vi "MPU_Stick_Generate_Emulator_Data.vi"() -> ()   [LabVIEW 2017]
uses:
  <vilib>/Utility/file.llb/Write Delimited Spreadsheet (string).vi
panel:
  in  "Step time (ms)":dbl=100.0
  in  "Number of samples":i32=100
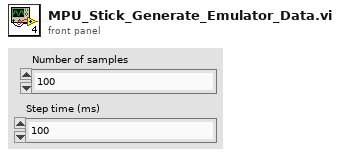
[diagram p1: front panel]
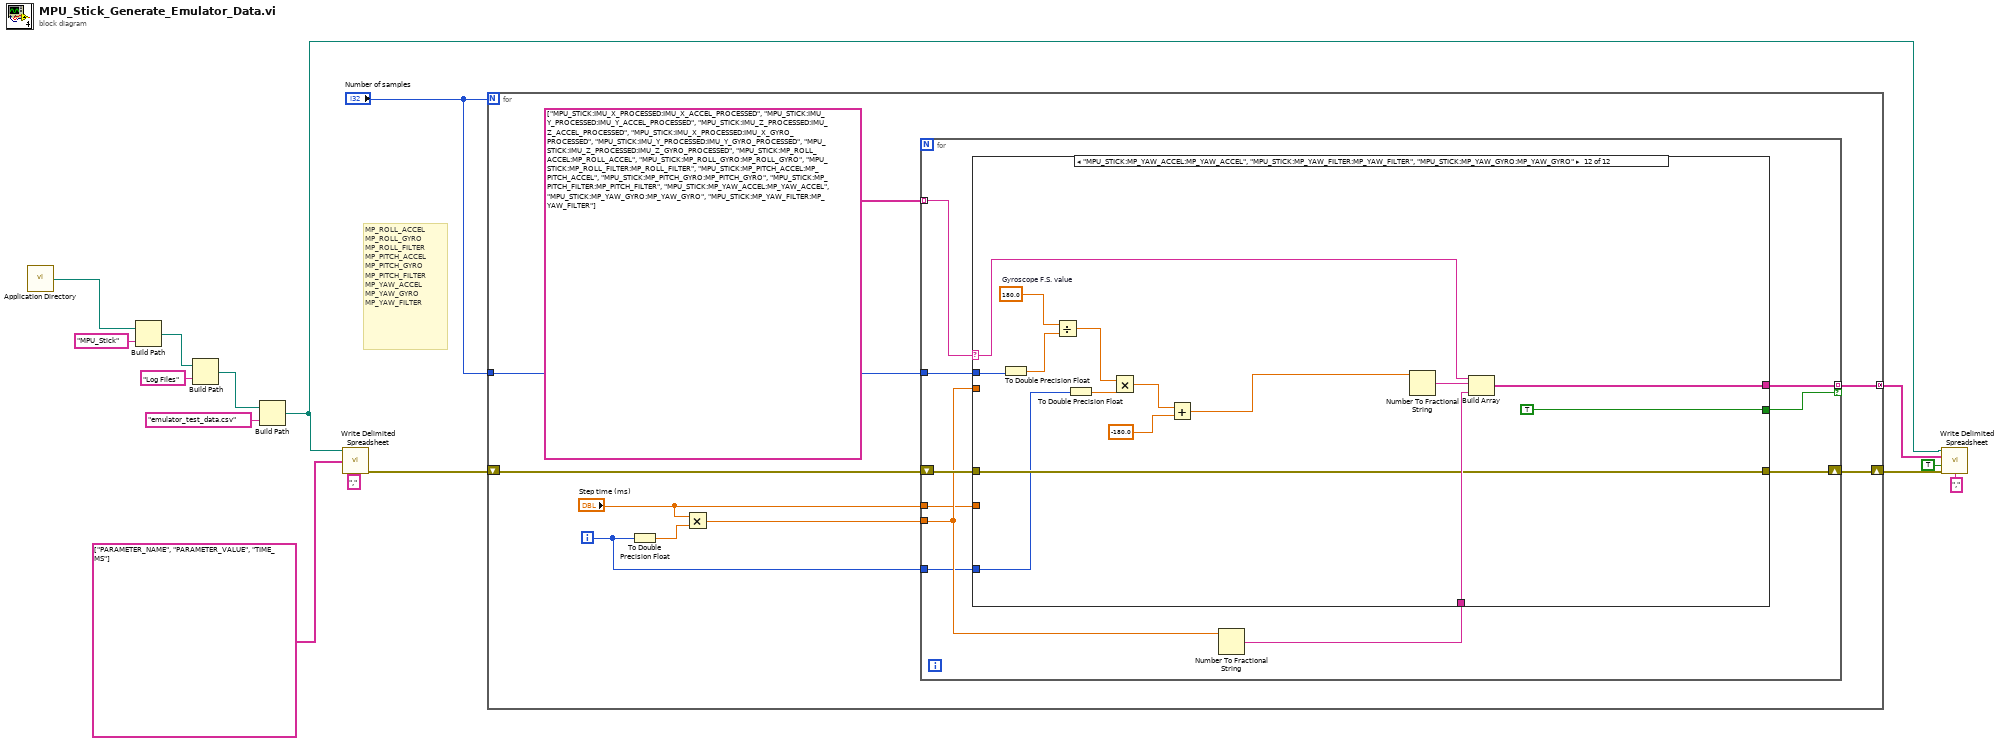
[diagram p0: block diagram]
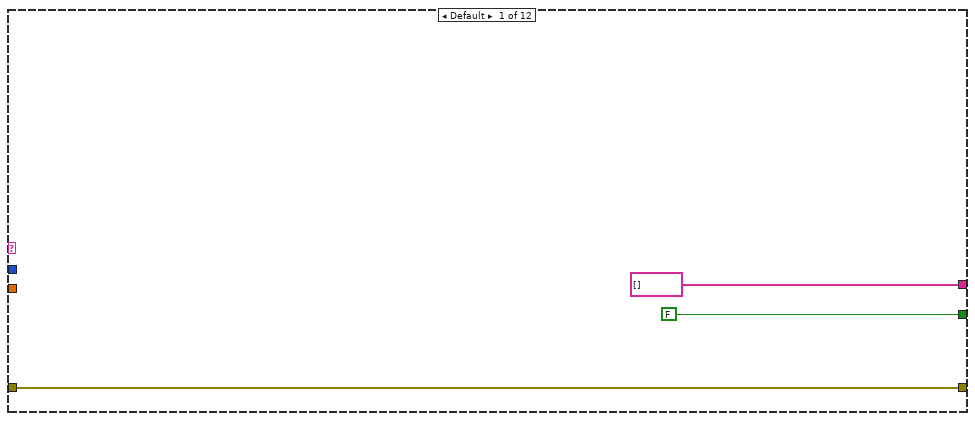
[diagram p2: hidden frame]
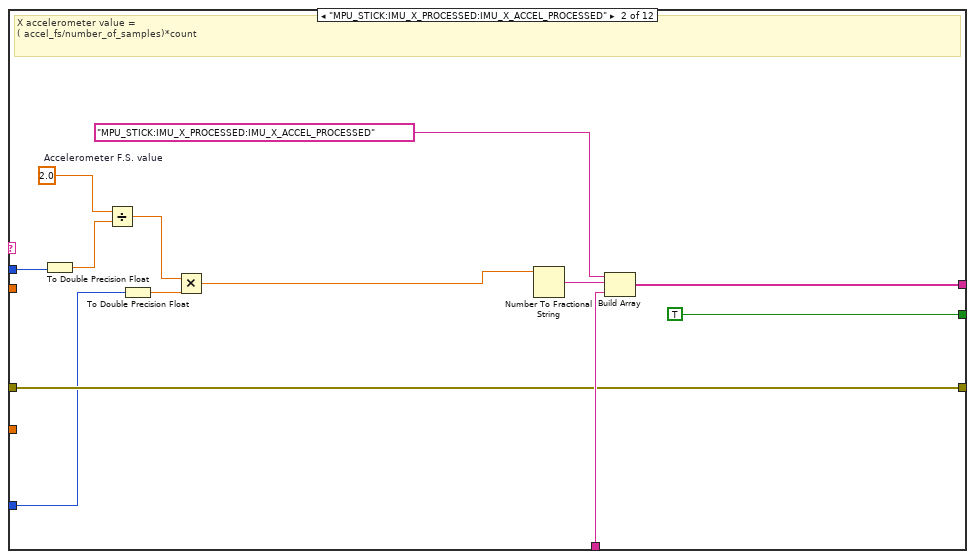
[diagram p3: hidden frame]
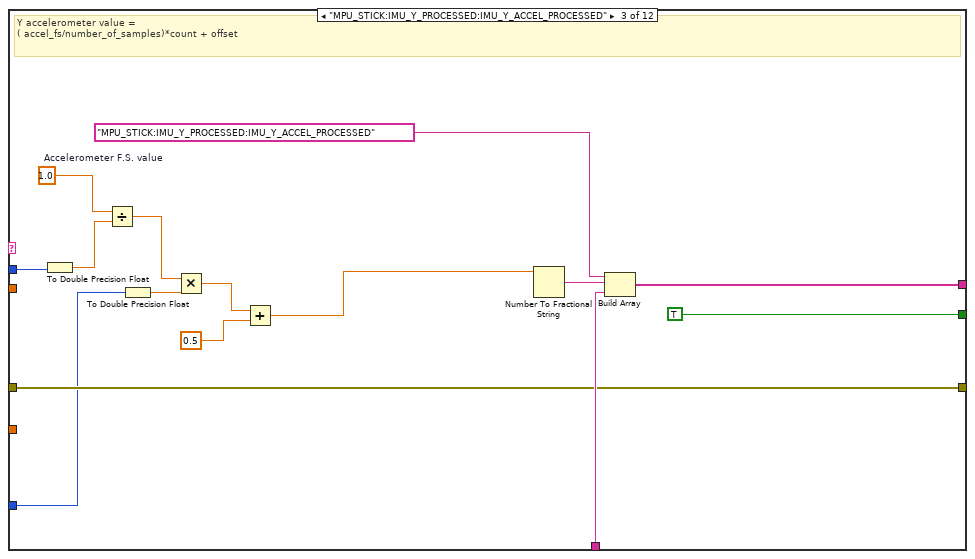
[diagram p4: hidden frame]
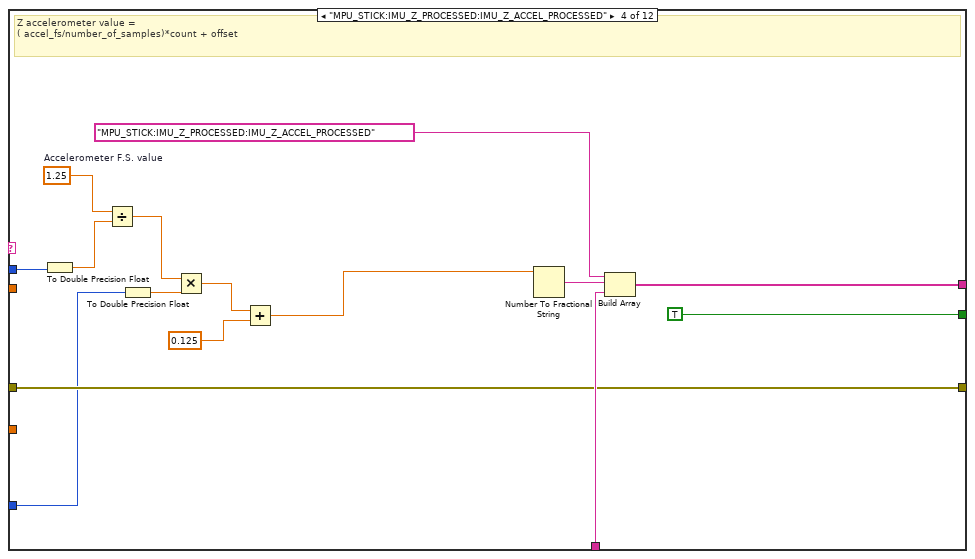
[diagram p5: hidden frame]
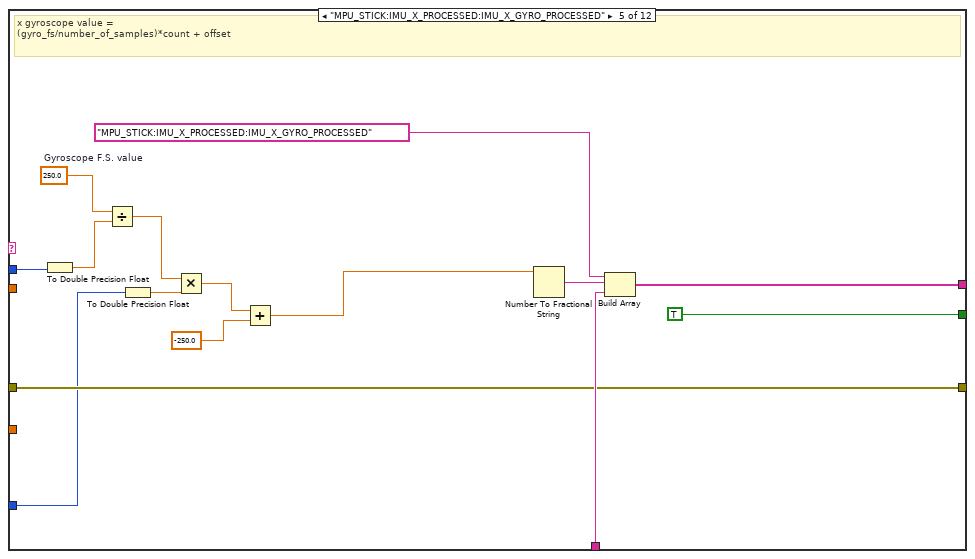
[diagram p6: hidden frame]
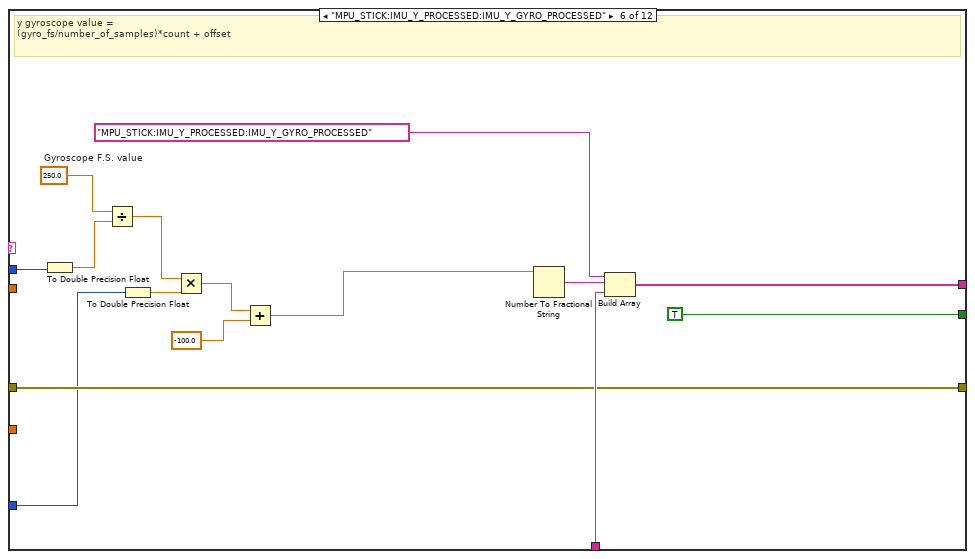
[diagram p7: hidden frame]
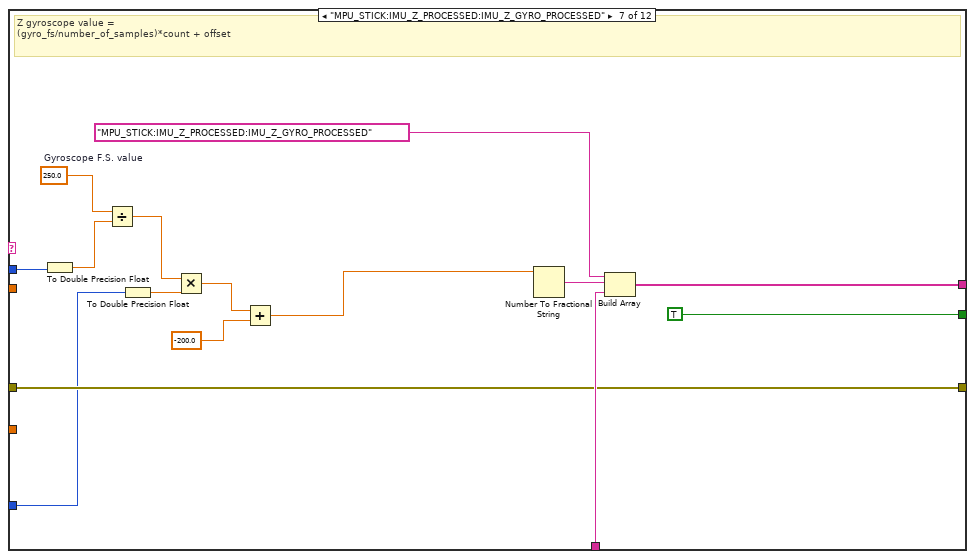
[diagram p8: hidden frame]
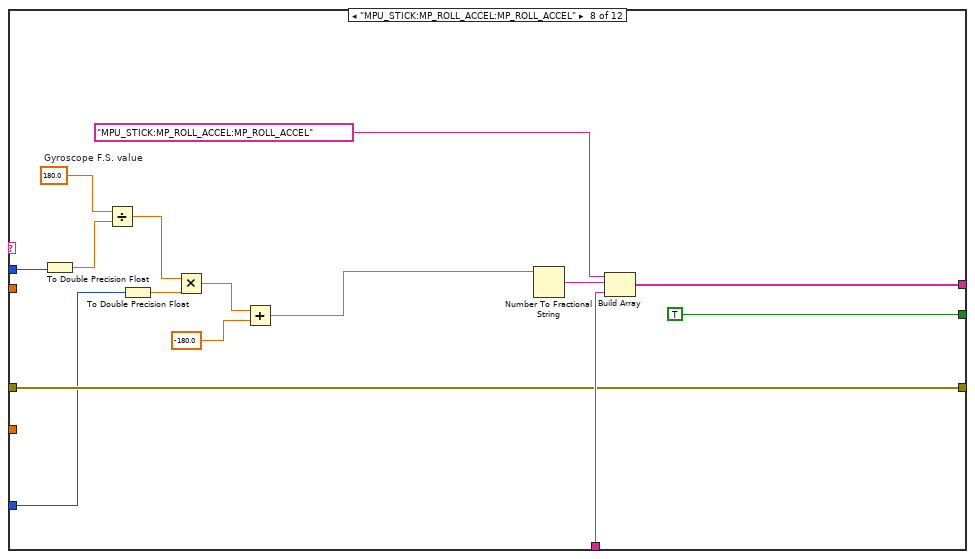
[diagram p9: hidden frame]
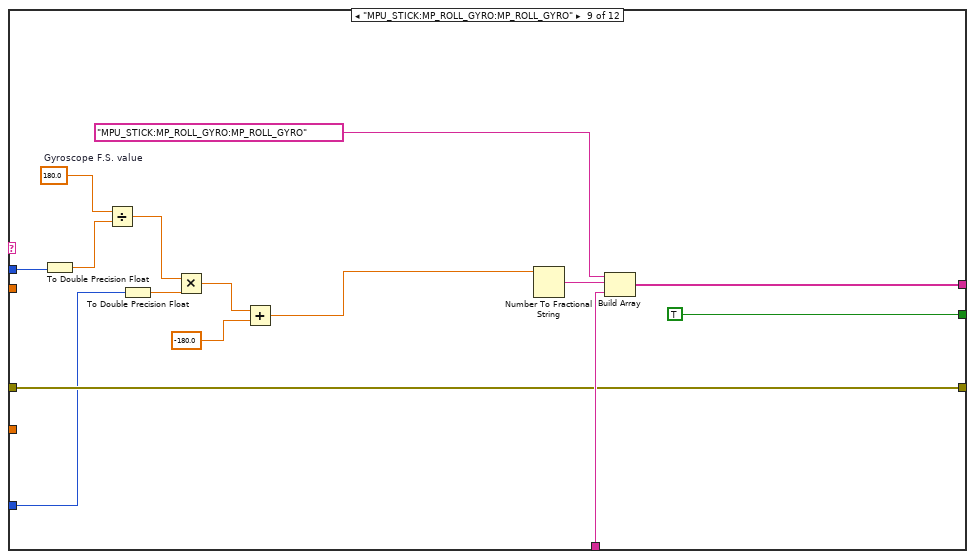
[diagram p10: hidden frame]
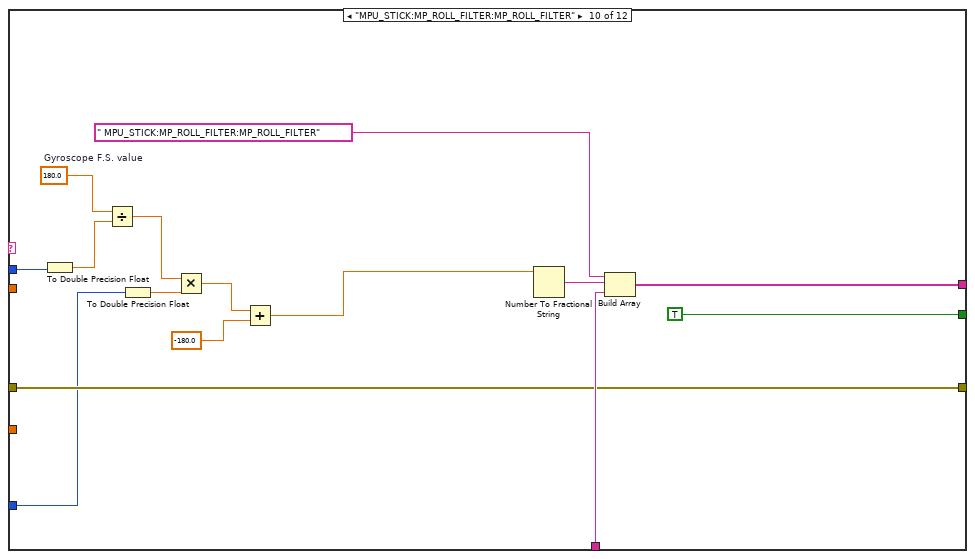
[diagram p11: hidden frame]
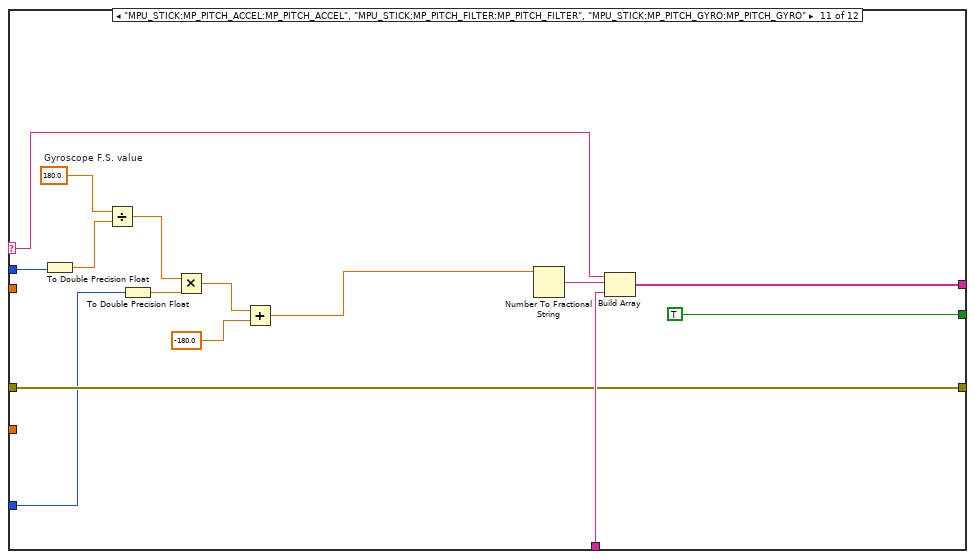
[diagram p12: hidden frame]
diagram:
  # "MP_ROLL_ACCEL\nMP_ROLL_GYRO\nMP_ROLL_FILTER\nMP_PITCH_ACCEL\nMP_PITCH_GYRO\nMP_PITCH_FILTER\nMP_YAW_ACCEL\nMP_YAW_GYRO\nMP_YAW_FILTER"
  n1 = call <vilib>:"Application Directory.vi"() -> ("Application Directory"=w10:path)
  n2 = Build Path(base path=w10, name or relative path="MPU_Stick") -> (appended path=w9:path)
  n3 = Build Path(base path=w9, name or relative path="Log Files") -> (appended path=w14:path)
  n4 = Build Path(base path=w14, name or relative path="emulator_test_data.csv") -> (appended path=w5:path)
  n5 = call-poly <vilib>:"Write Delimited Spreadsheet.vi"("file path (dialog if empty)"=w5, "1D data"=string[] ["PARAMETER_NAME", "PARAMETER_VALUE", "TIME_MS"], "delimiter (\\t)"="," ("delimiter (\\t)")) -> ("error out"=w7:errorcluster)  [unwired: 11 in, 1 out]
  n6 = for {
    N: "Number of samples" -> [_]
    shift-right: [w20] -> w6
    shift-left: w7 -> [w23]
    tunnel: [w17] -> w4 mode=concatenating
    tunnel: "Number of samples" -> [w16]
    i -> [w19]
    n7 = To Double Precision Float(number=w19) -> (double precision float=w22:dbl)
    n8 = Multiply(x="Step time (ms)", y=w22) -> (x*y=w21:dbl)
    n9 = for {
      tunnel: string[] ["MPU_STICK:IMU_X_PROCESSED:IMU_X_ACCEL_PROCESSED", "MPU_STICK:IMU_Y_PROCESSED:IMU_Y_ACCEL_PROCESSED", "MPU_STICK:IMU_Z_PROCESSED:IMU_Z_ACCEL_PROCESSED", "MPU_STICK:IMU_X_PROCESSED:IMU_X_GYRO_PROCESSED", "MPU_STICK:IMU_Y_PROCESSED:IMU_Y_GYRO_PROCESSED", "MPU_STICK:IMU_Z_PROCESSED:IMU_Z_GYRO_PROCESSED", "MPU_STICK:MP_ROLL_ACCEL:MP_ROLL_ACCEL", "MPU_STICK:MP_ROLL_GYRO:MP_ROLL_GYRO", "MPU_STICK:MP_ROLL_FILTER:MP_ROLL_FILTER", "MPU_STICK:MP_PITCH_ACCEL:MP_PITCH_ACCEL", "MPU_STICK:MP_PITCH_GYRO:MP_PITCH_GYRO", "MPU_STICK:MP_PITCH_FILTER:MP_PITCH_FILTER", "MPU_STICK:MP_YAW_ACCEL:MP_YAW_ACCEL", "MPU_STICK:MP_YAW_GYRO:MP_YAW_GYRO", "MPU_STICK:MP_YAW_FILTER:MP_YAW_FILTER"] -> [w33] mode=indexing
      tunnel: w21 -> [w31]
      shift-right: [w32] -> w20
      shift-left: w23 -> [w34]
      tunnel: w19 -> [w30]
      tunnel: "Step time (ms)" -> [w29]
      tunnel: [w27] -> w17 mode=indexing if=w26
      tunnel: w16 -> [w25]
      n10 = Number To Fractional String(number=w31) -> (F-format string=w28:string)  [unwired: 3 in]
      n11 = case shown="\"MPU_STICK:MP_YAW_ACCEL:MP_YAW_ACCEL\", \"MPU_STICK:MP_YAW_FILTER:MP_YAW_FILTER\", \"MPU_STICK:MP_YAW_GYRO:MP_YAW_GYRO\"" w33 {
        selector: w33 -> [_ _ _ _ _ _ _ _ _ _ w171 w186]
        tunnel: w34 -> [w37 w47 w62 w77 w92 w107 w122 w137 w152 w167 w183 w198]
        tunnel: [w37 w47 w62 w77 w92 w107 w122 w137 w152 w167 w183 w198] -> w32
        tunnel: w31 -> [_ _ _ _ _ _ _ _ _ _ _ _]
        tunnel: w30 -> [_ w40 w55 w70 w85 w100 w115 w130 w145 w160 w176 w191]
        tunnel: w29 -> [_ _ _ _ _ _ _ _ _ _ _ _]
        tunnel: w28 -> [_ w48 w63 w78 w93 w108 w123 w138 w153 w168 w184 w199]
        tunnel: [string[] [] w46 w61 w76 w91 w106 w121 w136 w151 w166 w182 w197] -> w27
        tunnel: [FALSE TRUE TRUE TRUE TRUE TRUE TRUE TRUE TRUE TRUE TRUE TRUE] -> w26
        tunnel: w25 -> [_ w43 w58 w73 w88 w103 w118 w133 w148 w163 w179 w194]
        frame Default {
        }
        frame "MPU_STICK:IMU_X_PROCESSED:IMU_X_ACCEL_PROCESSED" {
          w44 = 2.0  # Accelerometer F.S. value
          # "X accelerometer value =\n( accel_fs/number_of_samples)*count"
          n12 = To Double Precision Float(number=w43) -> (double precision float=w42:dbl)
          n13 = Divide(x=w44, y=w42) -> (x/y=w41:dbl)
          n14 = To Double Precision Float(number=w40) -> (double precision float=w39:dbl)
          n15 = Multiply(x=w41, y=w39) -> (x*y=w38:dbl)
          n16 = Number To Fractional String(number=w38) -> (F-format string=w50:string)  [unwired: 3 in]
          n17 = Build Array("MPU_STICK:IMU_X_PROCESSED:IMU_X_ACCEL_PROCESSED", w50, w48) -> (w46:string[])
        }
        frame "MPU_STICK:IMU_Y_PROCESSED:IMU_Y_ACCEL_PROCESSED" {
          w59 = 1.0  # Accelerometer F.S. value
          # "Y accelerometer value =\n( accel_fs/number_of_samples)*count + offset"
          n18 = To Double Precision Float(number=w58) -> (double precision float=w57:dbl)
          n19 = Divide(x=w59, y=w57) -> (x/y=w56:dbl)
          n20 = To Double Precision Float(number=w55) -> (double precision float=w54:dbl)
          n21 = Multiply(x=w56, y=w54) -> (x*y=w53:dbl)
          n22 = Add(x=w53, y=0.5) -> (x+y=w51:dbl)
          n23 = Number To Fractional String(number=w51) -> (F-format string=w65:string)  [unwired: 3 in]
          n24 = Build Array("MPU_STICK:IMU_Y_PROCESSED:IMU_Y_ACCEL_PROCESSED", w65, w63) -> (w61:string[])
        }
        frame "MPU_STICK:IMU_Z_PROCESSED:IMU_Z_ACCEL_PROCESSED" {
          w74 = 1.25  # Accelerometer F.S. value
          # "Z accelerometer value =\n( accel_fs/number_of_samples)*count + offset"
          n25 = To Double Precision Float(number=w73) -> (double precision float=w72:dbl)
          n26 = Divide(x=w74, y=w72) -> (x/y=w71:dbl)
          n27 = To Double Precision Float(number=w70) -> (double precision float=w69:dbl)
          n28 = Multiply(x=w71, y=w69) -> (x*y=w68:dbl)
          n29 = Add(x=w68, y=0.125) -> (x+y=w66:dbl)
          n30 = Number To Fractional String(number=w66) -> (F-format string=w80:string)  [unwired: 3 in]
          n31 = Build Array("MPU_STICK:IMU_Z_PROCESSED:IMU_Z_ACCEL_PROCESSED", w80, w78) -> (w76:string[])
        }
        frame "MPU_STICK:IMU_X_PROCESSED:IMU_X_GYRO_PROCESSED" {
          w89 = 250.0  # Gyroscope F.S. value
          # "x gyroscope value =\n(gyro_fs/number_of_samples)*count + offset"
          n32 = To Double Precision Float(number=w88) -> (double precision float=w87:dbl)
          n33 = Divide(x=w89, y=w87) -> (x/y=w86:dbl)
          n34 = To Double Precision Float(number=w85) -> (double precision float=w84:dbl)
          n35 = Multiply(x=w86, y=w84) -> (x*y=w83:dbl)
          n36 = Add(x=w83, y=-250.0) -> (x+y=w81:dbl)
          n37 = Number To Fractional String(number=w81) -> (F-format string=w95:string)  [unwired: 3 in]
          n38 = Build Array("MPU_STICK:IMU_X_PROCESSED:IMU_X_GYRO_PROCESSED", w95, w93) -> (w91:string[])
        }
        frame "MPU_STICK:IMU_Y_PROCESSED:IMU_Y_GYRO_PROCESSED" {
          w104 = 250.0  # Gyroscope F.S. value
          # "y gyroscope value =\n(gyro_fs/number_of_samples)*count + offset"
          n39 = To Double Precision Float(number=w103) -> (double precision float=w102:dbl)
          n40 = Divide(x=w104, y=w102) -> (x/y=w101:dbl)
          n41 = To Double Precision Float(number=w100) -> (double precision float=w99:dbl)
          n42 = Multiply(x=w101, y=w99) -> (x*y=w98:dbl)
          n43 = Add(x=w98, y=-100.0) -> (x+y=w96:dbl)
          n44 = Number To Fractional String(number=w96) -> (F-format string=w110:string)  [unwired: 3 in]
          n45 = Build Array("MPU_STICK:IMU_Y_PROCESSED:IMU_Y_GYRO_PROCESSED", w110, w108) -> (w106:string[])
        }
        frame "MPU_STICK:IMU_Z_PROCESSED:IMU_Z_GYRO_PROCESSED" {
          w119 = 250.0  # Gyroscope F.S. value
          # "Z gyroscope value =\n(gyro_fs/number_of_samples)*count + offset"
          n46 = To Double Precision Float(number=w118) -> (double precision float=w117:dbl)
          n47 = Divide(x=w119, y=w117) -> (x/y=w116:dbl)
          n48 = To Double Precision Float(number=w115) -> (double precision float=w114:dbl)
          n49 = Multiply(x=w116, y=w114) -> (x*y=w113:dbl)
          n50 = Add(x=w113, y=-200.0) -> (x+y=w111:dbl)
          n51 = Number To Fractional String(number=w111) -> (F-format string=w125:string)  [unwired: 3 in]
          n52 = Build Array("MPU_STICK:IMU_Z_PROCESSED:IMU_Z_GYRO_PROCESSED", w125, w123) -> (w121:string[])
        }
        frame "MPU_STICK:MP_ROLL_ACCEL:MP_ROLL_ACCEL" {
          w134 = 180.0  # Gyroscope F.S. value
          n53 = To Double Precision Float(number=w133) -> (double precision float=w132:dbl)
          n54 = Divide(x=w134, y=w132) -> (x/y=w131:dbl)
          n55 = To Double Precision Float(number=w130) -> (double precision float=w129:dbl)
          n56 = Multiply(x=w131, y=w129) -> (x*y=w128:dbl)
          n57 = Add(x=w128, y=-180.0) -> (x+y=w126:dbl)
          n58 = Number To Fractional String(number=w126) -> (F-format string=w140:string)  [unwired: 3 in]
          n59 = Build Array("MPU_STICK:MP_ROLL_ACCEL:MP_ROLL_ACCEL", w140, w138) -> (w136:string[])
        }
        frame "MPU_STICK:MP_ROLL_GYRO:MP_ROLL_GYRO" {
          w149 = 180.0  # Gyroscope F.S. value
          n60 = To Double Precision Float(number=w148) -> (double precision float=w147:dbl)
          n61 = Divide(x=w149, y=w147) -> (x/y=w146:dbl)
          n62 = To Double Precision Float(number=w145) -> (double precision float=w144:dbl)
          n63 = Multiply(x=w146, y=w144) -> (x*y=w143:dbl)
          n64 = Add(x=w143, y=-180.0) -> (x+y=w141:dbl)
          n65 = Number To Fractional String(number=w141) -> (F-format string=w155:string)  [unwired: 3 in]
          n66 = Build Array("MPU_STICK:MP_ROLL_GYRO:MP_ROLL_GYRO", w155, w153) -> (w151:string[])
        }
        frame "MPU_STICK:MP_ROLL_FILTER:MP_ROLL_FILTER" {
          w164 = 180.0  # Gyroscope F.S. value
          n67 = To Double Precision Float(number=w163) -> (double precision float=w162:dbl)
          n68 = Divide(x=w164, y=w162) -> (x/y=w161:dbl)
          n69 = To Double Precision Float(number=w160) -> (double precision float=w159:dbl)
          n70 = Multiply(x=w161, y=w159) -> (x*y=w158:dbl)
          n71 = Add(x=w158, y=-180.0) -> (x+y=w156:dbl)
          n72 = Number To Fractional String(number=w156) -> (F-format string=w170:string)  [unwired: 3 in]
          n73 = Build Array(" MPU_STICK:MP_ROLL_FILTER:MP_ROLL_FILTER", w170, w168) -> (w166:string[])
        }
        frame "MPU_STICK:MP_PITCH_ACCEL:MP_PITCH_ACCEL", "MPU_STICK:MP_PITCH_FILTER:MP_PITCH_FILTER", "MPU_STICK:MP_PITCH_GYRO:MP_PITCH_GYRO" {
          w180 = 180.0  # Gyroscope F.S. value
          n74 = To Double Precision Float(number=w179) -> (double precision float=w178:dbl)
          n75 = Divide(x=w180, y=w178) -> (x/y=w177:dbl)
          n76 = To Double Precision Float(number=w176) -> (double precision float=w175:dbl)
          n77 = Multiply(x=w177, y=w175) -> (x*y=w174:dbl)
          n78 = Add(x=w174, y=-180.0) -> (x+y=w172:dbl)
          n79 = Number To Fractional String(number=w172) -> (F-format string=w185:string)  [unwired: 3 in]
          n80 = Build Array(w171, w185, w184) -> (w182:string[])
        }
        frame "MPU_STICK:MP_YAW_ACCEL:MP_YAW_ACCEL", "MPU_STICK:MP_YAW_FILTER:MP_YAW_FILTER", "MPU_STICK:MP_YAW_GYRO:MP_YAW_GYRO" {
          w195 = 180.0  # Gyroscope F.S. value
          n81 = To Double Precision Float(number=w194) -> (double precision float=w193:dbl)
          n82 = Divide(x=w195, y=w193) -> (x/y=w192:dbl)
          n83 = To Double Precision Float(number=w191) -> (double precision float=w190:dbl)
          n84 = Multiply(x=w192, y=w190) -> (x*y=w189:dbl)
          n85 = Add(x=w189, y=-180.0) -> (x+y=w187:dbl)
          n86 = Number To Fractional String(number=w187) -> (F-format string=w200:string)  [unwired: 3 in]
          n87 = Build Array(w186, w200, w199) -> (w197:string[])
        }
      }
    }
  }
  n88 = call-poly <vilib>:"Write Delimited Spreadsheet.vi"("file path (dialog if empty)"=w5, "2D data"=w4, "append to file? (new file:F)"=TRUE, "error in (no error)"=w6, "delimiter (\\t)"="," ("delimiter (\\t)")) -> ()  [unwired: 9 in, 2 out]
